vi "Programatic Scroll.vi"(8 "error in":errorcluster, 9 "PauseResume Ref":refnum<vi>, 10 "Table Ref":refnum<vi>, 11 "Trace":string[][](table)=[["", "", "", "", ""], ["", "", "", "", ""], ["", "", "", "", ""], ["", "", "", "", ""], ["", "", "", "", ""], ["", "", "", "", ""]]) -> (0 "error out":errorcluster)   [LabVIEW 2025, in "CAN-LIN Raw Bus Capture UI.lvlib"]
doc: "Scroll the table programatically to the end (only necessary when it is unpaused, paused table will not get new data). This vi does this scrolling only when it is not paused."
uses:
  CAN-LIN Raw Bus Capture UI.lvlib
  <vilib>/Utility/miscctls.llb/LVRowAndColumnUnsignedTypeDef.ctl
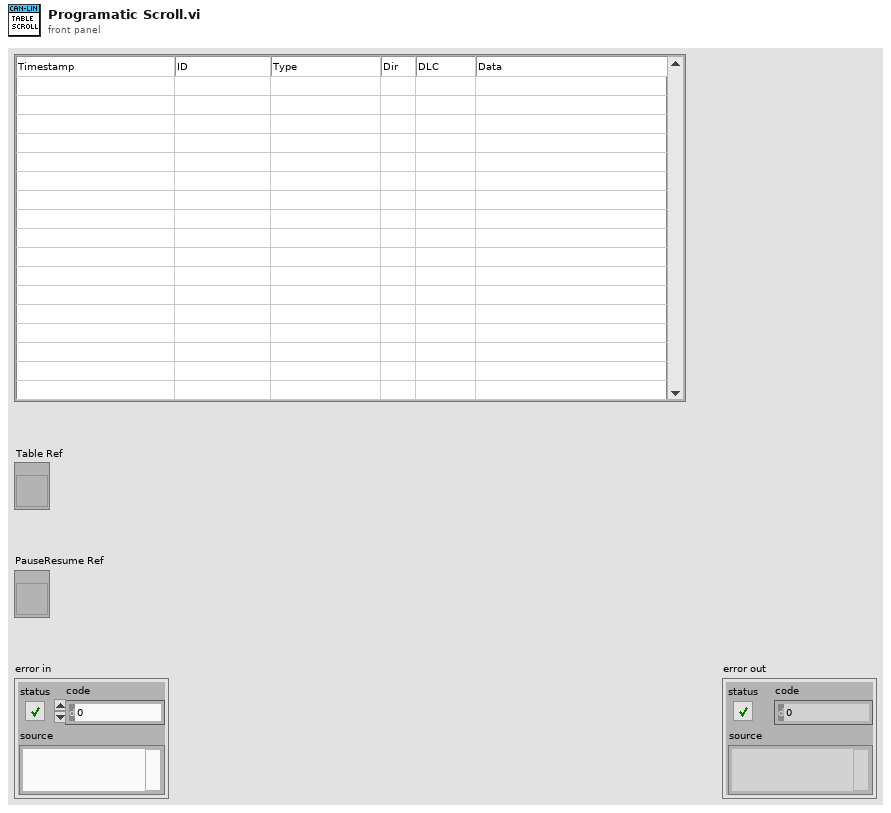
[diagram p1: front panel]
types:
  T1 = typedef "LVRowAndColumnUnsignedTypeDef.ctl" = cluster{"Row":u32, "Column":u32}
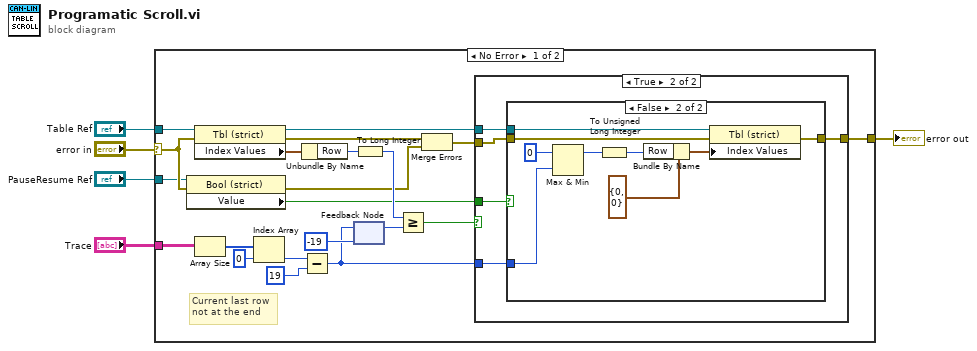
[diagram p0: block diagram]
diagram:
  n1 = case shown="No Error" "error in" {
    selector: "error in" -> [w11 w43]
    tunnel: "Table Ref" -> [w25 _]
    tunnel: "Trace" -> [w18 _]
    tunnel: [w26 w43] -> w3
    tunnel: "PauseResume Ref" -> [w10 _]
    frame No Error {
      # "Current last row\nnot at the end"
      n2 = property on="Property Node" class="Bool (strict)"(reference=w10, error in=w11) -> (error out=w9:errorcluster, "Value"=w6:bool)  [unwired: 1 out]
      n3 = property on="Property Node" class="Tbl (strict)"(reference=w25, error in=w11) -> (reference out=w24:refnum<vi>, error out=w8:errorcluster, "Index Values"=w23:T1)
      n4 = Array Size(array=w18) -> (size(s)=w21:i32[])
      n5 = Index Array(array=w21, index=0) -> (element=w22:i32)
      n6 = Unbundle By Name(w23) -> ("Row"=w15:u32)
      n7 = Subtract(x=w22, y=19 ("max(x,y)")) -> (x-y=w12:i32)
      n8 = feedback #1(-19 ("max(x,y)")) -> (w14:i32)
      n9 = feedback-in #1(w12) -> ()
      n10 = To Long Integer(number=w15) -> (32bit integer=w17:i32)
      n11 = Greater Or Equal?(x=w17, y=w14) -> (x >= y?=w16:bool)
      n12 = Merge Errors(w8, w9) -> (w7:errorcluster)
      n13 = case shown="True" w16 {
        tunnel: [w27 w32] -> w26
        tunnel: w24 -> [_ w31]
        tunnel: w7 -> [w27 w30]
        tunnel: w12 -> [_ w29]
        tunnel: w6 -> [_ w28]
        frame False {
        }
        frame True {
          n14 = case shown="False" w28 {
            tunnel: w31 -> [_ w42]
            tunnel: w30 -> [w33 w41]
            tunnel: [w33 w40] -> w32
            tunnel: w29 -> [_ w34]
            frame True {
            }
            frame False {
              n15 = Max & Min(x=0 ("max(x,y)"), y=w34) -> (max(x,y)=w36:i32)  [unwired: 1 out]
              n16 = To Unsigned Long Integer(number=w36) -> (unsigned 32bit integer=w35:u32)
              n17 = Bundle By Name(cluster=T1 {"Row"=0, "Column"=0} ("Index Values"), "Row"=w35) -> (w38:T1)
              n18 = property on="Property Node" class="Tbl (strict)"(reference=w42, error in=w41, "Index Values"=w38) -> (error out=w40:errorcluster)  [unwired: 1 out]
            }
          }
        }
      }
    }
    frame Error {
    }
  }
  "error out" <- w3
